vi "Initialize (Simulator).vi"(8 "error in (no error)":errorcluster, 10 "Z Index Enabled (F:Disable)":bool, 11 "Device ID":T1) -> (0 "error out":errorcluster, 3 "Maxon Encoder out":refnum<class "Maxon Encoder.lvclass">)   [LabVIEW 2019, in "Maxon Encoder Simulator.lvclass"]
doc: "Establishes communication with the sensor. Therefore, call this VI before calling other sensor driver VIs for this sensor. Generally, you need to call the Initialize VI only once at the beginning of an application."
uses:
  Maxon Encoder Simulator.lvclass
  Maxon Encoder.lvclass
  <vilib>/robotics/Simulator/NI_Robotics_Simulator.lvlib
  <vilib>/robotics/Simulator/Engine/ctl/DeviceID.ctl
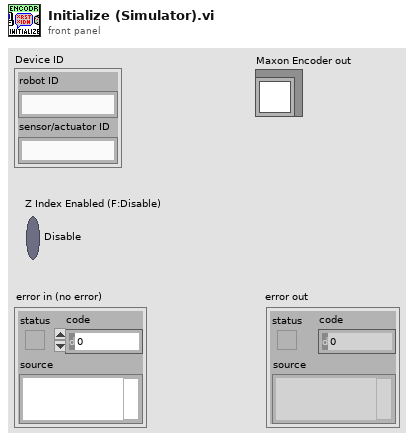
[diagram p1: front panel]
types:
  T1 = typedef "NI_Robotics_Simulator.lvlib/DeviceID.ctl" = cluster{"robot ID":string, "sensor/actuator ID":string}
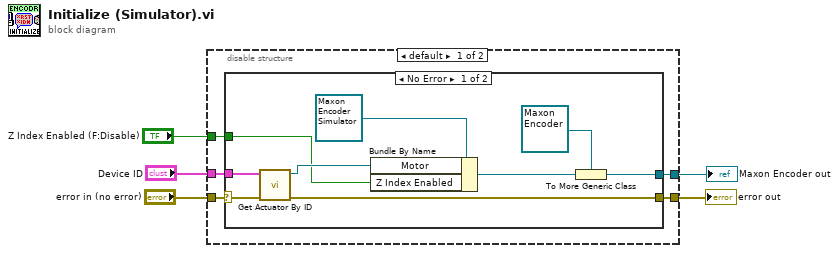
[diagram p0: block diagram]
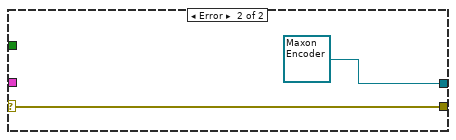
[diagram p2: hidden frame]
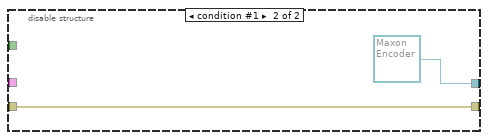
[diagram p3: hidden frame]
diagram:
  n1 = disable-structure shown="default" {
    disable-tunnel: "error in (no error)" -> [w10 w23]
    disable-tunnel: "Device ID" -> [w9 _]
    disable-tunnel: [w8 w23] -> w2
    disable-tunnel: [w7 refnum<class "Maxon Encoder.lvclass"> refnum ("Maxon Encoder.lvclass")] -> w4
    disable-tunnel: "Z Index Enabled (F:Disable)" -> [w6 _]
    frame condition #0 (active) {
      n2 = case shown="No Error" w10 {
        selector: w10 -> [w13 w21]
        tunnel: w9 -> [w15 _]
        tunnel: [w19 refnum<class "Maxon Encoder.lvclass"> refnum ("Maxon Encoder.lvclass")] -> w7
        tunnel: [w14 w21] -> w8
        tunnel: w6 -> [w11 _]
        frame No Error {
          n3 = call <vilib>:"Get Actuator By ID.vi"("error in (no error)"=w13, "device ID"=w15) -> ("error out"=w14:errorcluster, "actuator class"=w12:refnum<class "ODESimulator_Motor.lvclass">)  [unwired: 8 in]
          n4 = Bundle By Name(cluster=refnum<class "Maxon Encoder Simulator.lvclass"> refnum ("Maxcon Encoder Simulator.lvclass"), "Motor"=w12, "Z Index Enabled"=w11) -> (w18:refnum<class "Maxon Encoder Simulator.lvclass">)
          n5 = To More Generic Class(target class=refnum<class "Maxon Encoder.lvclass"> refnum ("Maxon Encoder.lvclass"), reference=w18) -> (generic class reference=w19:refnum<class "Maxon Encoder.lvclass">)
        }
        frame Error {
        }
      }
    }
    frame condition #1 {
    }
  }
  "error out" <- w2
  "Maxon Encoder out" <- w4
